vi "Calculate Color Index Array.vi"(8 "error in (no error)":errorcluster, 10 "3D Stem Datatype in":refnum<class "3D Stem Datatype.lvclass">, 11 "Plot Representation In":T1) -> (0 "error out":errorcluster, 2 "3D Stem Datatype out":refnum<class "3D Stem Datatype.lvclass">, 3 "Plot Representation Out":T1)   [LabVIEW 2017, in "3D Stem Datatype.lvclass"]
uses:
  <vilib>/Math Plots/3D Math Plots/3D Stem/3D Stem Datatype/3D Stem Datatype.lvclass
  <vilib>/Math Plots/3D Math Plots/3D Plot/3D Plot/Typedef/Plot Representation.ctl
  <vilib>/Math Plots/3D Math Plots/3D Plot/3D Plot/Typedef/Range Clusters.ctl
  <vilib>/Math Plots/3D Math Plots/3D Plot/3D Plot/Typedef/Mesh Data.ctl
  <vilib>/Math Plots/3D Math Plots/3D Stem/3D Stem Datatype/3D Stem Datatype.lvclass/3D Stem Datatype.ctl
  <vilib>/Math Plots/3D Math Plots/3D Plot/3D Plot Datatype/3D Plot Datatype.lvclass
  <vilib>/Math Plots/3D Math Plots/3D Plot/3D Plot/3D Plot.lvclass
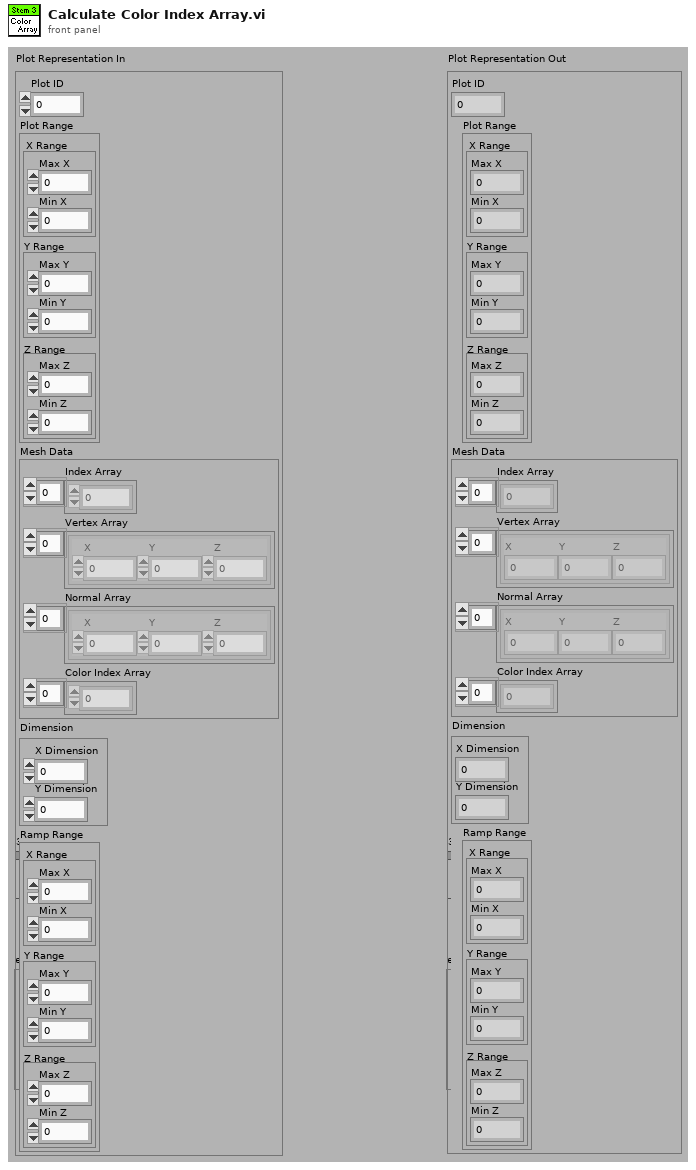
[diagram p1: front panel]
types:
  T1 = typedef "3D Plot.lvclass/Plot Representation.ctl" = cluster{"Plot ID":i32, "Plot Range":T2, "Mesh Data":T3, "Dimension":cluster{"X Dimension":i32, "Y Dimension":i32}, "Ramp Range":T2}
  T2 = typedef "3D Plot.lvclass/Range Clusters.ctl" = cluster{"X Range":cluster{"Max X":sgl, "Min X":sgl}, "Y Range":cluster{"Max Y":sgl, "Min Y":sgl}, "Z Range":cluster{"Max Z":sgl, "Min Z":sgl}}
  T3 = typedef "3D Plot.lvclass/Mesh Data.ctl" = cluster{"Index Array":u32[], "Vertex Array":cluster{"X":sgl, "Y":sgl, "Z":sgl}[], "Normal Array":cluster{"X":sgl, "Y":sgl, "Z":sgl}[], "Color Index Array":i32[]}
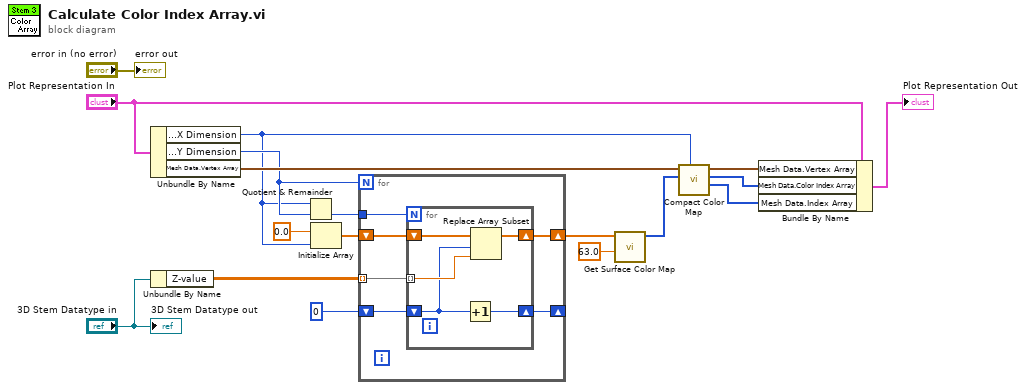
[diagram p0: block diagram]
diagram:
  n1 = Unbundle By Name("Plot Representation In") -> ("Dimension.X Dimension"=w1:i32, "Dimension.Y Dimension"=w3:i32, "Mesh Data.Vertex Array"=w10:cluster{"X":sgl, "Y":sgl, "Z":sgl}[])
  n2 = Unbundle By Name("3D Stem Datatype in") -> ("Z-value"=w6:sgl[][])
  n3 = Quotient & Remainder(x=w1, y=w3) -> (floor(x/y)=w2:i32)  [unwired: 1 out]
  n4 = Initialize Array(sgl 0.0 ("element"), w1) -> (w8:sgl[])
  n5 = for {
    N: w3 -> [_]
    tunnel: w2 -> [w24]
    shift-right: [w19] -> w5
    shift-left: w8 -> [w23]
    tunnel: w6 -> [w22] mode=indexing
    shift-right: [w21] -> _
    shift-left: 0 -> [w20]
    n6 = for {
      N: w24 -> [_]
      shift-right: [w28] -> w19
      shift-left: w23 -> [w29]
      tunnel: w22 -> [w27] mode=indexing
      shift-right: [w26] -> w21
      shift-left: w20 -> [w25]
      n7 = Increment(x=w25) -> (x+1=w26:i32)
      n8 = Replace Array Subset(array=w29, new element=w27, index=w25) -> (w28:sgl[])
    }
  }
  n9 = call <vilib>:"Get Surface Color Map.vi"("Levels"=sgl 63.0, "Amplifiy"=w5) -> ("Color Index Array"=w14:i32[])  [unwired: 9 out]
  n10 = call <vilib>:"Compact Color Map.vi"("X Dimension"=w1, "Color Index Array In"=w14, "Vertex Array In"=w10) -> ("Index for Same Color Vertex"=w11:u32[], "Compact Color Index Array Out"=w12:i32[], "Reordered Vertex Array Out"=w13:cluster{"X":sgl, "Y":sgl, "Z":sgl}[])  [unwired: 3 in, 3 out]
  n11 = Bundle By Name(cluster="Plot Representation In", "Mesh Data.Vertex Array"=w13, "Mesh Data.Color Index Array"=w12, "Mesh Data.Index Array"=w11) -> (→"Plot Representation Out":T1)
  "error out" <- "error in (no error)"
  "3D Stem Datatype out" <- "3D Stem Datatype in"
